vi "MessageMaker.vi"(1 "Power":i32, 2 "Output Port (All Ports)":T1=3 items=["Port A"=0, "Port B"=1, "Port C"=2, "Ports A & B"=4, "Ports A & C"=5, "Ports B & C"=6, "All Ports"=3], 3 "Port (Port 1)":T2 items=["Port 1", "Port 2", "Port 3", "Port 4"], 4 "R/W (T=R/F=W)":bool) -> (0 "Message":string)   [LabVIEW 2013]
uses:
  <vilib>/NXT/Block Support/NXT_InputPort.ctl
  <vilib>/NXT/Subs/MotorOutput.ctl
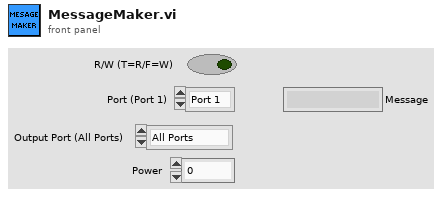
[diagram p1: front panel]
types:
  T1 = typedef "MotorOutput.ctl" = u8
  T2 = typedef "NXT_InputPort.ctl" = u32
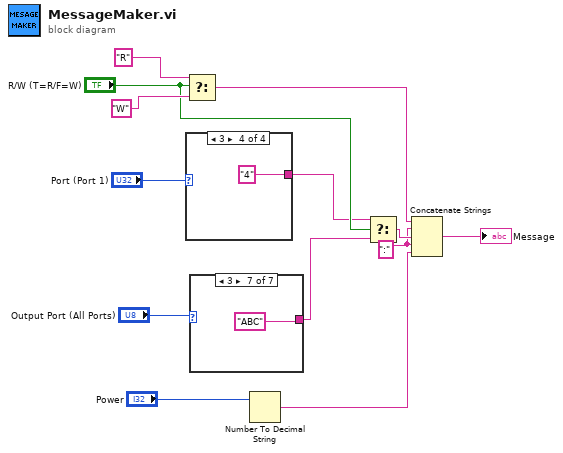
[diagram p0: block diagram]
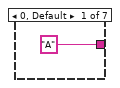
[diagram p2: hidden frame]
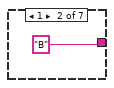
[diagram p3: hidden frame]
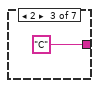
[diagram p4: hidden frame]
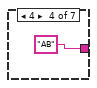
[diagram p5: hidden frame]
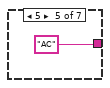
[diagram p6: hidden frame]
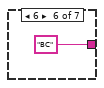
[diagram p7: hidden frame]
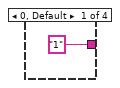
[diagram p8: hidden frame]
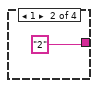
[diagram p9: hidden frame]
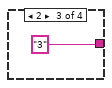
[diagram p10: hidden frame]
diagram:
  w1 = ":" ("string")
  n1 = case shown="3" "Port (Port 1)" {
    tunnel: ["1" "2" "3" "4"] -> w6
    frame 0, Default {
    }
    frame 1 {
    }
    frame 2 {
    }
    frame 3 {
    }
  }
  n2 = Select(t="R", s="R/W (T=R/F=W)", f="W") -> (s? t:f=w8:string)
  n3 = case shown="3" "Output Port (All Ports)" {
    tunnel: ["A" "B" "C" "AB" "AC" "BC" "ABC"] -> w5
    frame 0, Default {
    }
    frame 1 {
    }
    frame 2 {
    }
    frame 4 {
    }
    frame 5 {
    }
    frame 6 {
    }
    frame 3 {
    }
  }
  n4 = Number To Decimal String(number="Power") -> (decimal integer string=w3:string)  [unwired: 1 in]
  n5 = Select(t=w6, s="R/W (T=R/F=W)", f=w5) -> (s? t:f=w2:string)
  n6 = Concatenate Strings(w8, w1, w2, w1, w3) -> (→"Message":string)
